vi "FindLastDiscData.vi"(11 "DiscData":i64[](array[numeric])) -> (2 "ValueOfLastDiscData":i64, 3 "IndexOfLastDiscData":i32)   [LabVIEW 2023, in "2024_9.lvclass"]
uses:
  2024_9.lvclass
  2024_9.lvclass/2024_9.ctl
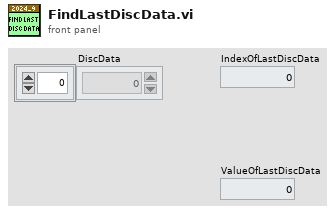
[diagram p1: front panel]
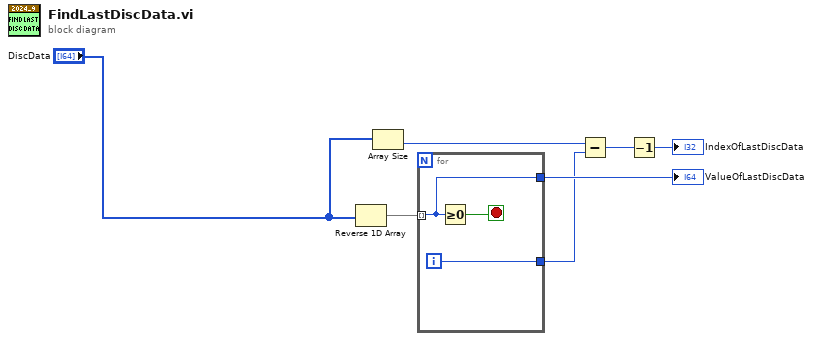
[diagram p0: block diagram]
diagram:
  n1 = Reverse 1D Array(array="DiscData") -> (reversed array=w2:i64[])
  n2 = Array Size(array="DiscData") -> (size(s)=w4:i32)
  n3 = for {
    tunnel: w2 -> [w8] mode=indexing
    tunnel: [w9] -> w5
    tunnel: [w8] -> w7
    i -> [w9]
    stop <- w10 stop-if-true
    n4 = Greater Or Equal To 0?(x=w8) -> (x >= 0?=w10:bool)
  }
  "ValueOfLastDiscData" <- w7
  n5 = Subtract(x=w4, y=w5) -> (x-y=w6:i32)
  n6 = Decrement(x=w6) -> (x-1=→"IndexOfLastDiscData":i32)
